vi "AlliGator Convert Decay Fit Parameter Constraints v2.vi"(8 "Error In":errorcluster, 10 "Fit Model":T3, 11 "Fit Parameter Constraints":T4[](array[typedef]) {"Max Value" format="%#.3g"; "Min Value" format="%#.3g"}) -> (0 "Error Out":errorcluster, 1 "Global Parameters?":bool[](array[boolean]), 3 "All Parameter Constraints":T1)   [LabVIEW 2021, in "AlliGator Decay Analysis.lvlib" / "AlliGator Decay Fit.lvlib"]
doc: "Returns constraints for all parameters of the model, even if the user only specified a few (or none at all).\n\nThis VI assumes that the <B>Fit Parameter Constraints</B> involve tau, and returns values with the same assumption.\n\nLook for constrained parameters. If present, replace default constraints (-Inf, Inf) by new ones, except for the offset, which is set to the guessed value (or zero if not provided)."
uses:
  AlliGator Decay Fit.lvlib
  AlliGator Decay Fit Parameter Constraints 2.ctl
  Fits/IRF(X)PSED/Decay Fit Parameters In List.ctl
  Fits/Decay Convolution/Decay Model.ctl
  Fits/IRF(X)PSED/Decay Fit Parameter Constraints Arrays.ctl
  Fits/Fits.lvlib
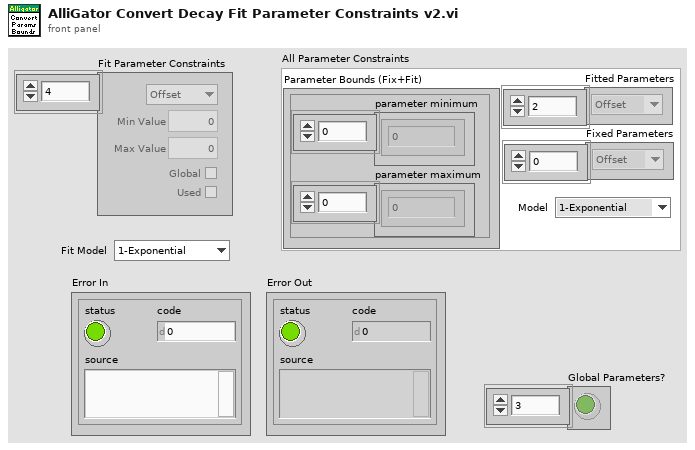
[diagram p1: front panel]
types:
  T1 = typedef "Fits.lvlib/Decay Fit Parameter Constraints Arrays.ctl" = cluster{"Parameter Bounds (Fix+Fit)":cluster{"parameter minimum":dbl[], "parameter maximum":dbl[]}, "Fitted Parameters":T2[], "Fixed Parameters":T2[], "Fit Model":T3}
  T2 = typedef "Fits.lvlib/Decay Fit Parameters In List.ctl" = enum16{"Offset", "Baseline", "A_1", "tau_1", "A_2", "tau_2"}
  T3 = typedef "Fits.lvlib/Decay Model.ctl" = enum16{"1-Exponential", "2-Exponentials"}
  T4 = typedef "AlliGator Decay Analysis.lvlib/AlliGator Decay Fit.lvlib/AlliGator Decay Fit Parameter Constraints 2.ctl" = cluster{"Fit Parameter":T2, "Min Value":dbl, "Max Value":dbl, "Global":bool, "Used":bool}
  T5 = cluster{"parameter minimum":dbl[], "parameter maximum":dbl[]}
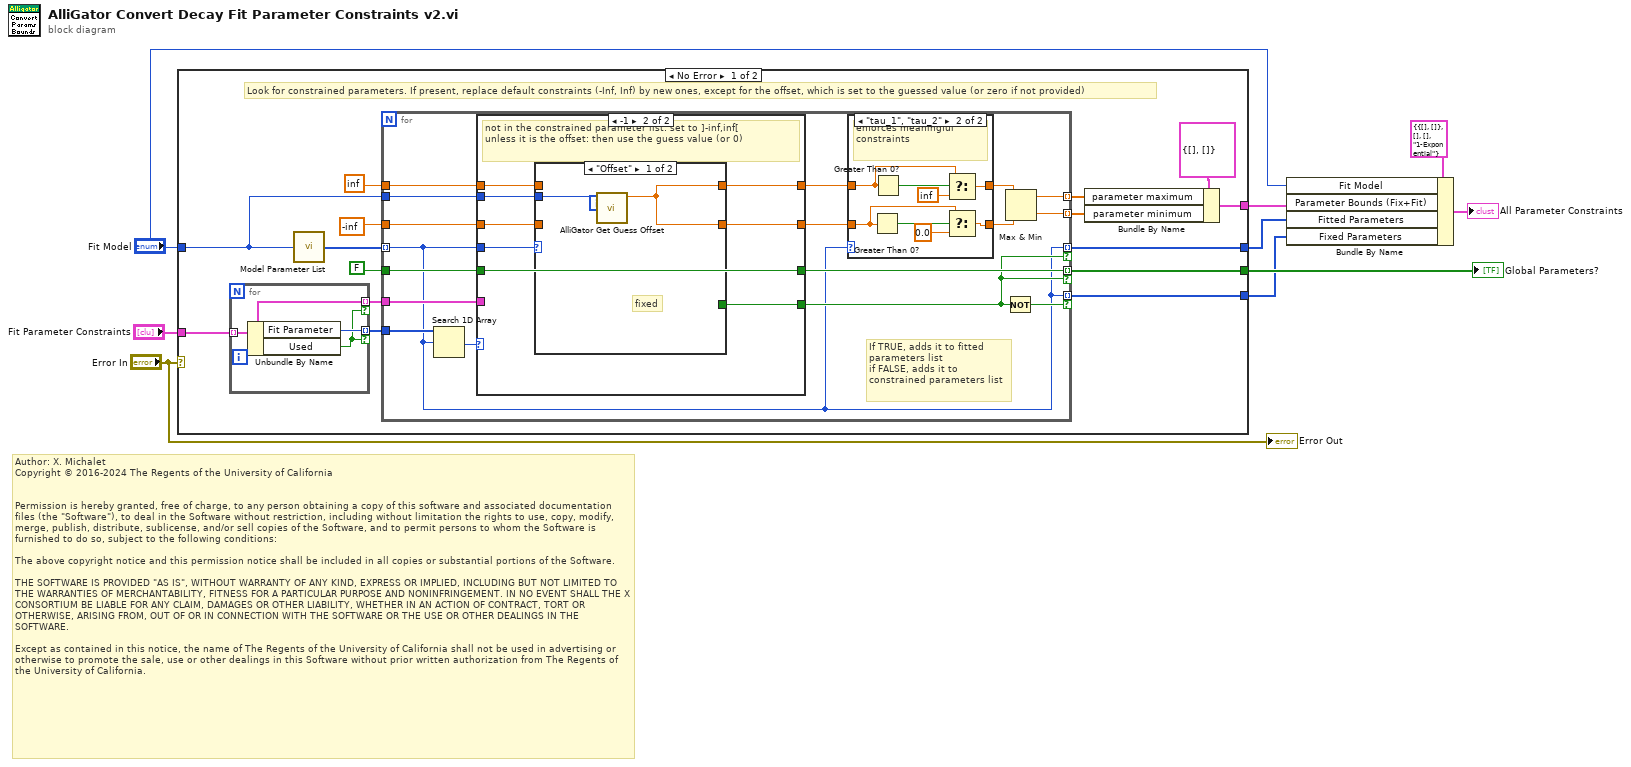
[diagram p0: block diagram]
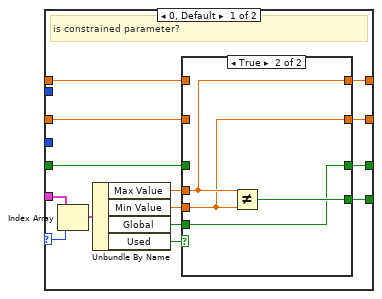
[diagram p3: hidden frame]
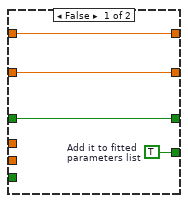
[diagram p4: hidden frame]
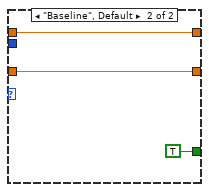
[diagram p5: hidden frame]
diagram:
  # "Author: X. Michalet\nCopyright © 2016-2024 The Regents of the University of California\n \n\nPermission is hereby granted, free of charge, to any person obtaining a copy of this software and associated documentation files (the \"Software\"), to deal in the Software without restriction, including without limitation the rights to use, copy, modify, merge, publish, distribute, sublicense, and/or sell copies of the Software, and to permit persons to whom the Software is furnished to do so, subject to the following conditions:\n\nThe above copyright notice and this permission notice shall be included in all copies or substantial portions of the Software.\n\nTHE SOFTWARE IS PROVIDED \"AS IS\", WITHOUT WARRANTY OF ANY KIND, EXPRESS OR IMPLIED, INCLUDING BUT NOT LIMITED TO THE WARRANTIES OF MERCHANTABILITY, FITNESS FOR A PARTICULAR PURPOSE AND NONINFRINGEMENT. IN NO EVENT SHALL THE X CONSORTIUM BE LIABLE FOR ANY CLAIM, DAMAGES OR OTHER LIABILITY, WHETHER IN AN ACTION OF CONTRACT, TORT OR OTHERWISE, ARISING FROM, OUT OF OR IN CONNECTION WITH THE SOFTWARE OR THE USE OR OTHER DEALINGS IN THE SOFTWARE.\n\nExcept as contained in this notice, the name of The Regents of the University of California shall not be used in advertising or otherwise to promote the sale, use or other dealings in this Software without prior written authorization from The Regents of the University of California."
  n1 = case shown="No Error" "Error In" {
    tunnel: "Fit Parameter Constraints" -> [w22 _]
    tunnel: [w20 _] -> w6
    tunnel: "Fit Model" -> [w10 _]
    tunnel: [w19 _] -> w7
    tunnel: [w15 _] -> w5
    tunnel: [w14 _] -> w4
    frame No Error {
      # "Look for constrained parameters. If present, replace default constraints (-Inf, Inf) by new ones, except for the offset, which is set to the guessed value (or zero if not provided)"
      n2 = for {
        tunnel: w22 -> [w88] mode=indexing
        tunnel: [w89] -> w24 mode=indexing if=w87
        tunnel: [w88] -> w13 mode=indexing if=w87
        n3 = Unbundle By Name(w88) -> ("Fit Parameter"=w89:T2, "Used"=w87:bool)
      }
      n4 = call "Model Parameter List.vi"("Fit Model"=w10) -> ("Model Parameter List"=w23:T2[])
      n5 = for {
        tunnel: w23 -> [w25] mode=indexing
        tunnel: w24 -> [w41]
        tunnel: w13 -> [w38]
        tunnel: inf ("element") -> [w40]
        tunnel: -inf ("element") -> [w39]
        tunnel: FALSE ("Global") -> [w37]
        tunnel: [w36] -> w19 mode=indexing if=w34
        tunnel: [w25] -> w15 mode=indexing if=w34
        tunnel: [w25] -> w14 mode=indexing if=w33
        tunnel: [w29] -> w12 mode=indexing
        tunnel: [w27] -> w11 mode=indexing
        tunnel: w10 -> [w26]
        # "If TRUE, adds it to fitted parameters list\nif FALSE, adds it to constrained parameters list"
        n6 = Search 1D Array(1D array=w41, element=w25) -> (index of element=w35:i32)  [unwired: 1 in]
        n7 = case shown="-1" w35 {
          selector: w35 -> [w65 _]
          tunnel: w40 -> [w62 w79]
          tunnel: [w57 w77] -> w32
          tunnel: w39 -> [w60 w78]
          tunnel: [w58 w76] -> w31
          tunnel: w38 -> [w64 _]
          tunnel: [w55 w81] -> w36
          tunnel: w37 -> [w56 w81]
          tunnel: [w52 w74] -> w34
          tunnel: w25 -> [_ w80]
          tunnel: w26 -> [_ w75]
          frame 0, Default {
            # "is constrained parameter?"
            n8 = Index Array(array=w64, index=w65) -> (element=w63:T4)
            n9 = Unbundle By Name(w63) -> ("Max Value"=w61:dbl, "Min Value"=w59:dbl, "Global"=w54:bool, "Used"=w53:bool)
            n10 = case shown="True" w53 {
              tunnel: w62 -> [w69 _]
              tunnel: w61 -> [_ w72]
              tunnel: w60 -> [w68 _]
              tunnel: w59 -> [_ w71]
              tunnel: [w68 w71] -> w58
              tunnel: [w69 w72] -> w57
              tunnel: w56 -> [w67 _]
              tunnel: [w67 w70] -> w55
              tunnel: w54 -> [_ w70]
              tunnel: [w66 w73] -> w52
              frame False {
                w66 = TRUE  # Add it to fitted parameters list
              }
              frame True {
                n11 = Not Equal?(x=w72, y=w71) -> (x != y?=w73:bool)
              }
            }
          }
          frame -1 {
            # "not in the constrained parameter list: set to ]-inf,inf[\nunless it is the offset: then use the guess value (or 0)"
            n12 = case shown="\"Offset\"" w80 {
              tunnel: w79 -> [_ w86]
              tunnel: w78 -> [_ w85]
              tunnel: [w82 w86] -> w77
              tunnel: [w82 w85] -> w76
              tunnel: w75 -> [w83 _]
              tunnel: [_ TRUE] -> w74
              frame "Offset" {
                # "fixed"
                n13 = call "AlliGator Get Guess Offset.vi"("Fit Model"=w83) -> ("Guess Offset"=w82:dbl)  [unwired: 9 in, 1 out]
              }
              frame "Baseline", Default {
              }
            }
          }
        }
        n14 = case shown="\"tau_1\", \"tau_2\"" w25 {
          tunnel: w32 -> [w43 w49]
          tunnel: w31 -> [w42 w51]
          tunnel: [w43 w48] -> w30
          tunnel: [w42 w50] -> w28
          frame "Offset", Default {
            # "Could potentially be -inf, +inf"
          }
          frame "tau_1", "tau_2" {
            # "enforces meaningful constraints"
            n15 = Greater Than 0?(x=w51) -> (x > 0?=w47:bool)
            n16 = Greater Than 0?(x=w49) -> (x > 0?=w46:bool)
            n17 = Select(t=w49, s=w46, f=inf) -> (s? t:f=w48:dbl)
            n18 = Select(t=w51, s=w47, f=0.0) -> (s? t:f=w50:dbl)
          }
        }
        n19 = Not(x=w34) -> (.not. x?=w33:bool)
        n20 = Max & Min(x=w30, y=w28) -> (max(x,y)=w29:dbl, min(x,y)=w27:dbl)
      }
      n21 = Bundle By Name(cluster=T5 {"parameter minimum"=[], "parameter maximum"=[]} ("parameter bounds"), "parameter maximum"=w12, "parameter minimum"=w11) -> (w20:T5)
    }
    frame Error {
    }
  }
  "Global Parameters?" <- w7
  n22 = Bundle By Name(cluster=T1 {"Parameter Bounds (Fix+Fit)"={"parameter minimum"=[], "parameter maximum"=[]}, "Fitted Parameters"=[], "Fixed Parameters"=[], "Fit Model"=enum."1-Exponential"} ("Parameter Constraints"), "Fit Model"="Fit Model", "Parameter Bounds (Fix+Fit)"=w6, "Fitted Parameters"=w5, "Fixed Parameters"=w4) -> (→"All Parameter Constraints":T1)
  "Error Out" <- "Error In"
